vi "Oscilloscope.vi"() -> ()   [LabVIEW 2018]
doc: "This is a PC based 8-Channel Oscilloscope designed as a virtual instrument. The hardware interface is developed using Arduino Nano.\n\n\nDeveloped by:\nTanmay Vilas Samak\nChinmay Vilas Samak"
uses:
  <vilib>/MakerHub/LINX/Public/Peripherals/Analog/Analog Read 1 Chan.vi
  <vilib>/MakerHub/LINX/Public/Peripherals/Analog/Analog Read N Chans.vi
  <vilib>/MakerHub/LINX/Private/Local IO/LinxAnalogRead.vi
  <vilib>/MakerHub/LINX/Public/Utilities/Check Channel.vi
  <vilib>/MakerHub/LINX/Public/Utilities/Open Serial.vi
  <vilib>/MakerHub/LINX/Private/Utilties/Generate Error.vi
  <vilib>/MakerHub/LINX/LMH-LINX.lvlib
panel:
  out "CH8":bool
  out "CH7":bool
  out "CH6":bool
  out "CH5":bool
  out "CH4":bool
  out "CH3":bool
  out "CH2":bool
  out "CH1":bool
  in  "CH8":bool
  in  "CH7":bool
  in  "PAUSE":bool
  in  "Radio Buttons":T1(radio)
  in  "Save Image Button":bool
  in  "File Type":T1(radio)
  in  "Record & Stop Button":bool
  out "Record Time":dbl
  in  "Serial Port":refnum<visa-resource-name>="N/A"
  in  "POWER":bool
  in  "VOLTAGE DIVISION":i32(knob) scale=0.0..4.0
  in  "TIME DIVISION":i32(knob) scale=0.0..4.0
  in  "CH6":bool
  in  "CH5":bool
  in  "CH4":bool
  in  "CH3":bool
  in  "CH2":bool
  in  "CH1":bool
  out "Oscilloscope":T2(graph)
  # "OSCILLOSCOPE"
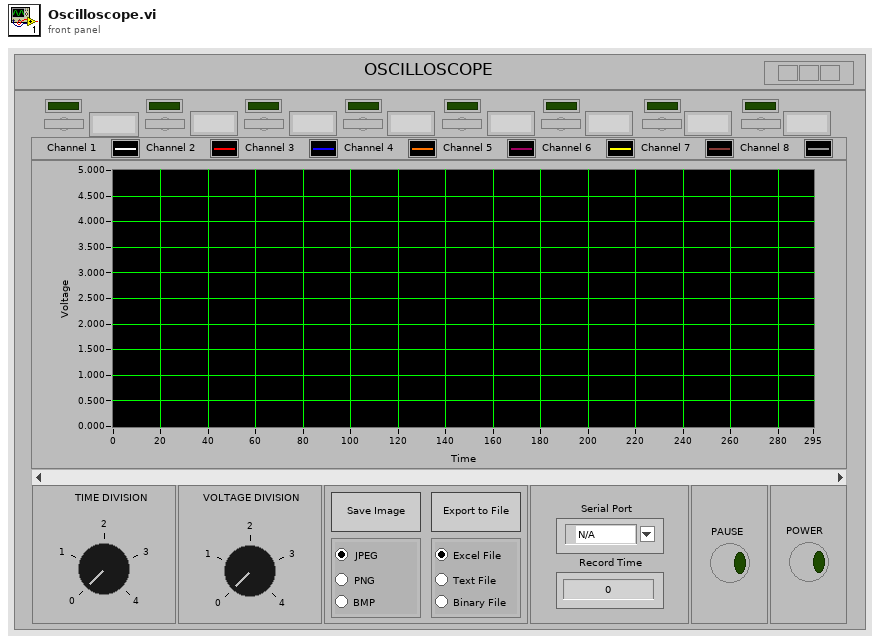
[diagram p1: front panel]
types:
  T1 = enum32{"Radio Selection 1", "Radio Selection 2", "Radio Selection 3"}
  T2 = cluster{"Voltage":dbl, "Voltage":dbl, "Voltage":dbl, "Voltage":dbl, "Voltage":dbl, "Voltage":dbl, "Voltage":dbl, "Voltage":dbl}
  T3 = cluster{"Voltage":dbl, "Voltage":dbl, "Voltage":dbl, "Voltage":dbl, "Voltage":dbl, "Voltage":dbl, "Voltage":dbl, "Voltage":dbl}[]
  T4 = enum8{"Enabled", "Disabled", "Disabled and Grayed Out"}
  T5 = typedef "LMH-LINX.lvlib/LINX Ref.ctl" = cluster{"IO":T6, "Interface":T7, "LINX Device Config":T8}
  T6 = typedef "LMH-LINX.lvlib/Platform.ctl" = enum16{"Remote", "Local"}
  T7 = typedef "LMH-LINX.lvlib/Interface.ctl" = enum16{"Serial", "TCP"}
  T8 = typedef "LMH-LINX.lvlib/Device.lvlib/LINX Device Config.ctl" = cluster{"Interface":T7, "COM Port":refnum<visa-resource-name>, "TCP Configuration":T9, "Device Family":u8, "Device ID":u8, "Device Name":string, "TCP Ref":refnum<k5>, "Channels":T10}
  T9 = typedef "LMH-LINX.lvlib/Device.lvlib/TCP Config.ctl" = cluster{"IP Address":string, "Port":u16}
  T10 = typedef "LMH-LINX.lvlib/Channels.ctl" = cluster{"DI":u8[], "DO":u8[], "AI":u8[], "AO":u8[], "PWM":u8[], "QE":u8[], "UART":u8[], "I2C 2":u8[], "SPI":u8[], "CAN":u8[], "Servo":u8[], "AI Ref (V)":dbl, "AI Resolution (Bits)":u8, "AO Ref (V)":dbl, "AO Resolution (Bits)":u8}
  T11 = typedef "imagedata.ctl" = cluster{"image type":i32, "image depth":i32, "image":u8[], "mask":u8[], "colors":u32[], "Rectangle":cluster{"left":i16, "top":i16, "right":i16, "bottom":i16}}
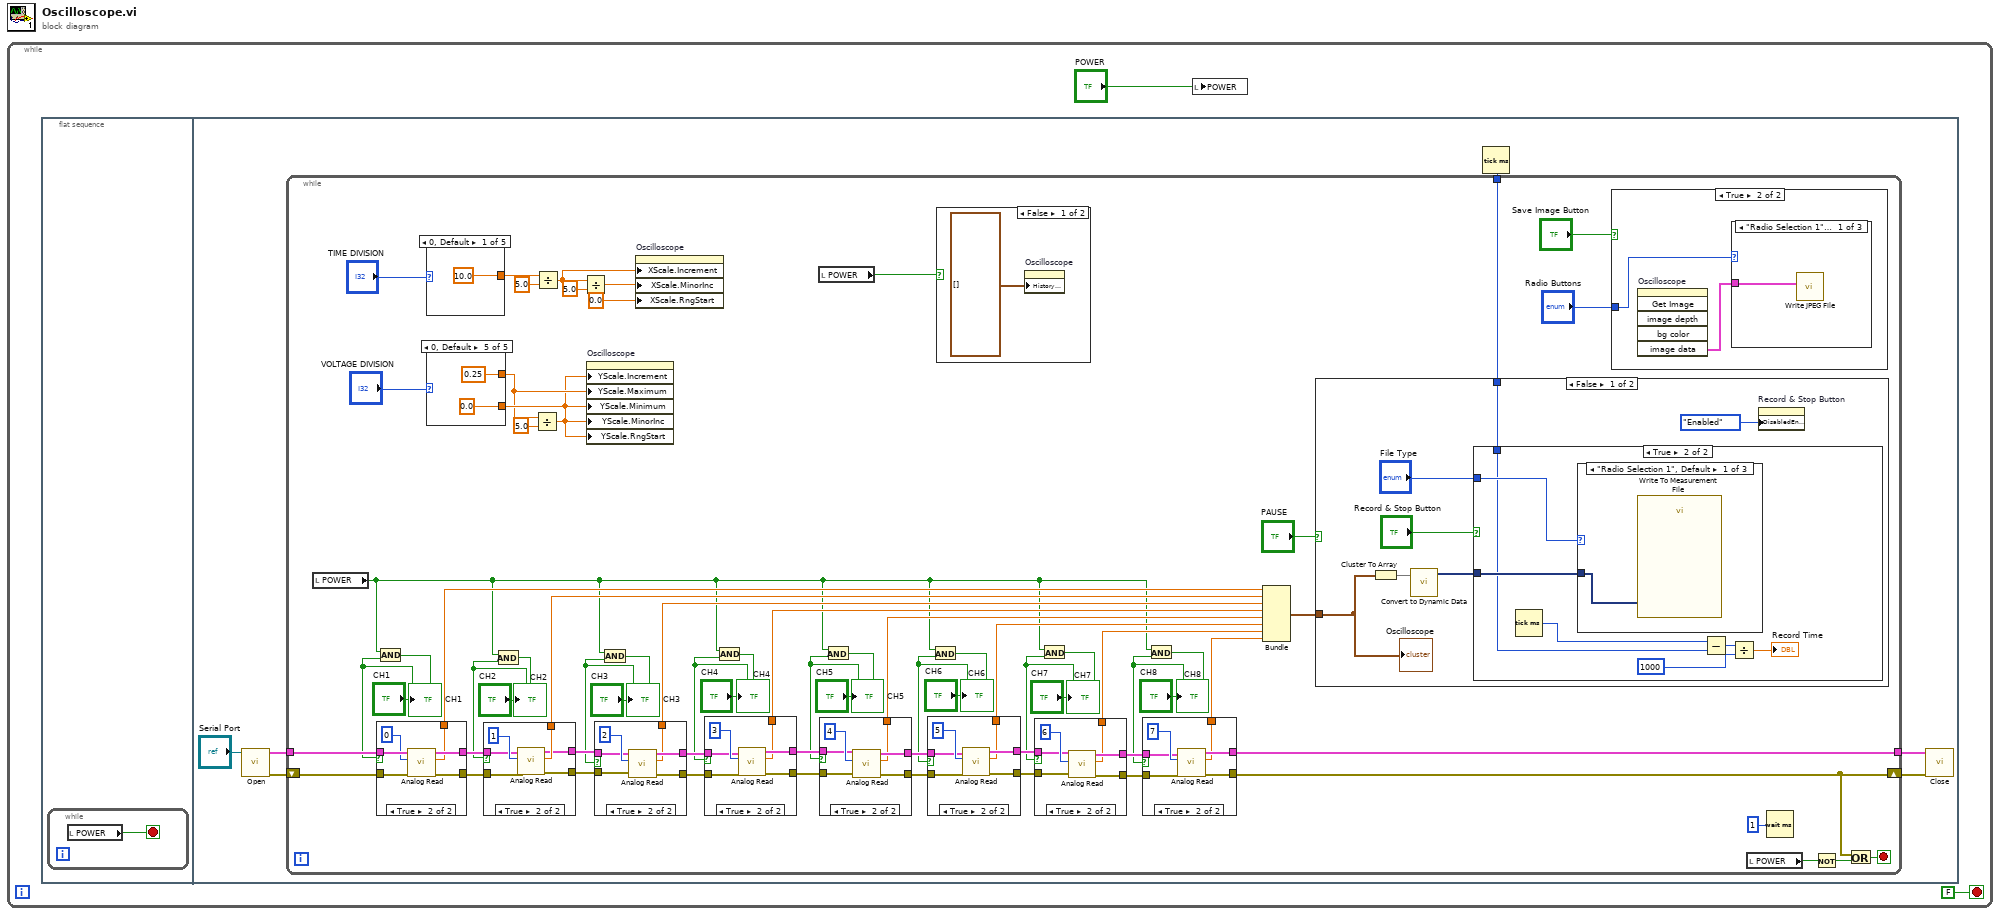
[diagram p0: block diagram]
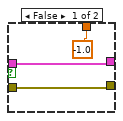
[diagram p3: hidden frame]
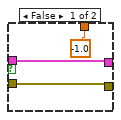
[diagram p4: hidden frame]
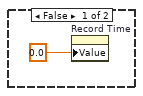
[diagram p5: hidden frame]
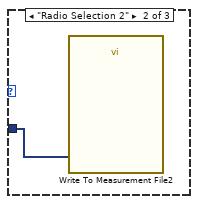
[diagram p6: hidden frame]
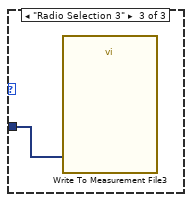
[diagram p7: hidden frame]
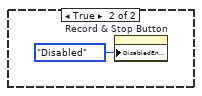
[diagram p8: hidden frame]
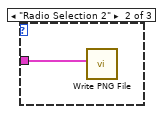
[diagram p10: hidden frame]
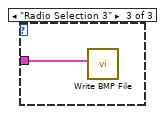
[diagram p11: hidden frame]
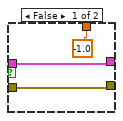
[diagram p12: hidden frame]
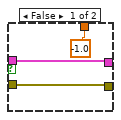
[diagram p13: hidden frame]
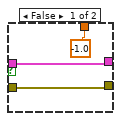
[diagram p14: hidden frame]
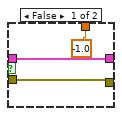
[diagram p15: hidden frame]
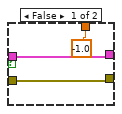
[diagram p16: hidden frame]
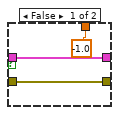
[diagram p17: hidden frame]
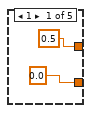
[diagram p18: hidden frame]
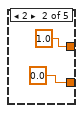
[diagram p19: hidden frame]
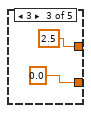
[diagram p20: hidden frame]
diagram:
  n1 = while {
    stop <- FALSE stop-if-true
    n2 = flat-sequence {
      frame #0 {
        n3 = while {
          stop <- w3 stop-if-true
          n4 = local read "POWER"() -> (w3:bool)
        }
      }
      frame #1 {
        n5 = call-poly <vilib>:"Open.vi"("Serial Port"="Serial Port") -> ("Error Out"=w7:errorcluster, "LINX Resource"=w6:T5)  [unwired: 8 in, 1 out]
        n6 = Tick Count (ms)() -> (millisecond timer value=w4:u32)
        n7 = while {
          shift-right: [w31] -> w9
          shift-left: w7 -> [w71]
          tunnel: w6 -> [w72]
          tunnel: [w32] -> w8
          tunnel: w4 -> [w38]
          stop <- w73 stop-if-true
          n8 = local read "POWER"() -> (w10:bool)
          n9 = case shown="True" "CH1" {
            tunnel: w72 -> [w165 w171]
            tunnel: w71 -> [w164 w170]
            tunnel: [w165 w168] -> w57
            tunnel: [w164 w167] -> w56
            tunnel: [-1.0 ("Voltage") w166] -> w55
            frame False {
            }
            frame True {
              n10 = call-poly <vilib>:"Analog Read.vi"("Error In"=w170, "Analog Channel"=u8 0 ("Channel 1 Pin"), "LINX Resource"=w171) -> ("Error Out"=w167:errorcluster, "Voltage"=w166:dbl, "LINX Resource"=w168:T5)  [unwired: 5 in, 1 out]
            }
          }
          n11 = And(x=w10, y="CH1") -> (x .and. y?=→"CH1":bool)
          n12 = case shown="0, Default" "TIME DIVISION" {
            tunnel: [10.0 20.0 50.0 100.0 200.0] -> w60
            frame 0, Default {
            }
            frame 1 {
            }
            frame 2 {
            }
            frame 3 {
            }
            frame 4 {
            }
          }
          n13 = case shown="0, Default" "VOLTAGE DIVISION" {
            tunnel: [0.5 1.0 2.5 5.0 0.25] -> w67
            tunnel: [0.0 0.0 0.0 0.0 0.0] -> w68
            frame 1 {
            }
            frame 2 {
            }
            frame 3 {
            }
            frame 4 {
            }
            frame 0, Default {
            }
          }
          n14 = case shown="True" "CH2" {
            tunnel: w57 -> [w155 w161]
            tunnel: w56 -> [w156 w160]
            tunnel: [-1.0 ("Voltage") w159] -> w54
            tunnel: [w156 w158] -> w51
            tunnel: [w155 w157] -> w42
            frame False {
            }
            frame True {
              n15 = call-poly <vilib>:"Analog Read.vi"("Error In"=w160, "Analog Channel"=u8 1 ("Channel 2 Pin"), "LINX Resource"=w161) -> ("Error Out"=w158:errorcluster, "Voltage"=w159:dbl, "LINX Resource"=w157:T5)  [unwired: 5 in, 1 out]
            }
          }
          n16 = And(x=w10, y="CH2") -> (x .and. y?=→"CH2":bool)
          n17 = Divide(x=w67, y=5.0) -> (x/y=w66:dbl)
          n18 = Divide(x=w60, y=5.0) -> (x/y=w62:dbl)
          n19 = Divide(x=w62, y=5.0) -> (x/y=w59:dbl)
          n20 = property on="Oscilloscope" class="WFChart (strict)"("YScale.Increment"=w66, "YScale.Maximum"=w67, "YScale.Minimum"=w68, "YScale.MinorInc"=w66, "YScale.RngStart"=w68) -> ()  [unwired: 2 in, 2 out]
          n21 = case shown="True" "CH3" {
            tunnel: [w147 w152] -> w53
            tunnel: [w146 w151] -> w52
            tunnel: w42 -> [w147 w150]
            tunnel: w51 -> [w146 w149]
            tunnel: [-1.0 ("Voltage") w148] -> w46
            frame False {
            }
            frame True {
              n22 = call-poly <vilib>:"Analog Read.vi"("Error In"=w149, "Analog Channel"=u8 2 ("Channel 3 Pin"), "LINX Resource"=w150) -> ("Error Out"=w151:errorcluster, "Voltage"=w148:dbl, "LINX Resource"=w152:T5)  [unwired: 5 in, 1 out]
            }
          }
          n23 = And(x=w10, y="CH3") -> (x .and. y?=→"CH3":bool)
          n24 = property on="Oscilloscope" class="WFChart (strict)"("XScale.Increment"=w62, "XScale.MinorInc"=w59, "XScale.RngStart"=0.0 ("X Scale.Range:Minimum")) -> ()  [unwired: 2 in, 2 out]
          n25 = case shown="True" "CH4" {
            tunnel: w53 -> [w138 w143]
            tunnel: w52 -> [w137 w142]
            tunnel: [w138 w141] -> w48
            tunnel: [w137 w140] -> w47
            tunnel: [-1.0 ("Voltage") w139] -> w45
            frame False {
            }
            frame True {
              n26 = call-poly <vilib>:"Analog Read.vi"("Error In"=w142, "Analog Channel"=u8 3 ("Channel 4 Pin"), "LINX Resource"=w143) -> ("Error Out"=w140:errorcluster, "Voltage"=w139:dbl, "LINX Resource"=w141:T5)  [unwired: 5 in, 1 out]
            }
          }
          n27 = And(x=w10, y="CH4") -> (x .and. y?=→"CH4":bool)
          n28 = local read "POWER"() -> (w25:bool)
          n29 = case shown="True" "CH5" {
            tunnel: [w129 w134] -> w50
            tunnel: [w128 w133] -> w49
            tunnel: w48 -> [w129 w132]
            tunnel: w47 -> [w128 w131]
            tunnel: [-1.0 ("Voltage") w130] -> w44
            frame False {
            }
            frame True {
              n30 = call-poly <vilib>:"Analog Read.vi"("Error In"=w131, "Analog Channel"=u8 4 ("Channel 5 Pin"), "LINX Resource"=w132) -> ("Error Out"=w133:errorcluster, "Voltage"=w130:dbl, "LINX Resource"=w134:T5)  [unwired: 5 in, 1 out]
            }
          }
          n31 = And(x=w10, y="CH5") -> (x .and. y?=→"CH5":bool)
          n32 = case shown="True" "CH6" {
            tunnel: w50 -> [w120 w125]
            tunnel: w49 -> [w119 w124]
            tunnel: [w120 w123] -> w34
            tunnel: [w119 w122] -> w33
            tunnel: [-1.0 ("Voltage") w121] -> w43
            frame False {
            }
            frame True {
              n33 = call-poly <vilib>:"Analog Read.vi"("Error In"=w124, "Analog Channel"=u8 5 ("Channel 6 Pin"), "LINX Resource"=w125) -> ("Error Out"=w122:errorcluster, "Voltage"=w121:dbl, "LINX Resource"=w123:T5)  [unwired: 5 in, 1 out]
            }
          }
          n34 = And(x=w10, y="CH6") -> (x .and. y?=→"CH6":bool)
          n35 = case shown="False" w25 {
            frame False {
              n36 = property on="Oscilloscope" class="WFChart (strict)"("History Data"=T3 []) -> ()  [unwired: 2 in, 2 out]
            }
            frame True {
            }
          }
          n37 = case shown="True" "CH7" {
            tunnel: [w87 w92] -> w36
            tunnel: [w86 w91] -> w35
            tunnel: w34 -> [w87 w90]
            tunnel: w33 -> [w86 w89]
            tunnel: [-1.0 ("Voltage") w88] -> w30
            frame False {
            }
            frame True {
              n38 = call-poly <vilib>:"Analog Read.vi"("Error In"=w89, "Analog Channel"=u8 6 ("Channel 5 Pin"), "LINX Resource"=w90) -> ("Error Out"=w91:errorcluster, "Voltage"=w88:dbl, "LINX Resource"=w92:T5)  [unwired: 5 in, 1 out]
            }
          }
          n39 = And(x=w10, y="CH7") -> (x .and. y?=→"CH7":bool)
          n40 = case shown="True" "CH8" {
            tunnel: w36 -> [w78 w83]
            tunnel: w35 -> [w77 w82]
            tunnel: [w78 w81] -> w32
            tunnel: [w77 w80] -> w31
            tunnel: [-1.0 ("Voltage") w79] -> w29
            frame False {
            }
            frame True {
              n41 = call-poly <vilib>:"Analog Read.vi"("Error In"=w82, "Analog Channel"=u8 7 ("Channel 6 Pin"), "LINX Resource"=w83) -> ("Error Out"=w80:errorcluster, "Voltage"=w79:dbl, "LINX Resource"=w81:T5)  [unwired: 5 in, 1 out]
            }
          }
          n42 = And(x=w10, y="CH8") -> (x .and. y?=→"CH8":bool)
          n43 = Bundle("Voltage"=w55, "Voltage"=w54, "Voltage"=w46, "Voltage"=w45, "Voltage"=w44, "Voltage"=w43, "Voltage"=w30, "Voltage"=w29) -> (w41:T2)  [unwired: 1 in]
          n44 = case shown="False" "PAUSE" {
            tunnel: w41 -> [w95 _]
            tunnel: w38 -> [w96 _]
            frame False {
              n45 = Cluster To Array(cluster=w95) -> (array=w97:dbl[])
              n46 = call "Convert to Dynamic Data"("Array"=w97) -> ("Dynamic Data Type"=w100:dynamicdata)  [unwired: 3 in]
              n47 = case shown="True" "Record & Stop Button" {
                tunnel: w100 -> [_ w108]
                tunnel: w96 -> [_ w102]
                tunnel: "File Type" -> [_ w104]
                frame False {
                  n48 = property on="Record Time" class="DigNum (strict)"("Value"=0.0 ("Recorded time")) -> ()  [unwired: 2 in, 2 out]
                }
                frame True {
                  n49 = Tick Count (ms)() -> (millisecond timer value=w103:u32)
                  n50 = case shown="\"Radio Selection 1\", Default" w104 {
                    tunnel: w108 -> [w109 w110 w111]
                    frame "Radio Selection 1", Default {
                      n51 = call "Write To Measurement File"("Signals"=w109) -> ()  [unwired: 16 in, 3 out]
                    }
                    frame "Radio Selection 2" {
                      n52 = call "Write To Measurement File2"("Signals"=w110) -> ()  [unwired: 16 in, 3 out]
                    }
                    frame "Radio Selection 3" {
                      n53 = call "Write To Measurement File3"("Signals"=w111) -> ()  [unwired: 16 in, 3 out]
                    }
                  }
                  n54 = Subtract(x=w103, y=w102) -> (x-y=w107:u32)
                  n55 = Divide(x=w107, y=u32 1000) -> (x/y=→"Record Time":dbl)
                }
              }
              n56 = property on="Record & Stop Button" class="Bool (strict)"("DisabledEnum"=T4."Enabled" ("Disabled")) -> ()  [unwired: 2 in, 2 out]
              "Oscilloscope" <- w95
            }
            frame True {
              n57 = property on="Record & Stop Button" class="Bool (strict)"("DisabledEnum"=T4."Disabled" ("Disabled")) -> ()  [unwired: 2 in, 2 out]
            }
          }
          n58 = case shown="True" "Save Image Button" {
            tunnel: "Radio Buttons" -> [_ w113]
            frame False {
            }
            frame True {
              n59 = invoke on="Oscilloscope" class="WFChart (strict)" method="Get Image"() -> ("image data"=w114:T11)  [unwired: 6 in, 5 out]
              n60 = case shown="\"Radio Selection 1\", Default" w113 {
                tunnel: w114 -> [w115 w116 w117]
                frame "Radio Selection 1", Default {
                  n61 = call <vilib>:"Write JPEG File.vi"("image data"=w115) -> ()  [unwired: 9 in, 2 out]
                }
                frame "Radio Selection 2" {
                  n62 = call <vilib>:"Write PNG File.vi"("image data"=w116) -> ()  [unwired: 9 in, 2 out]
                }
                frame "Radio Selection 3" {
                  n63 = call <vilib>:"Write BMP File.vi"("image data"=w117) -> ()  [unwired: 9 in, 2 out]
                }
              }
            }
          }
          n64 = local read "POWER"() -> (w28:bool)
          n65 = Wait (ms)(milliseconds to wait=u32 1) -> ()  [unwired: 1 out]
          n66 = Not(x=w28) -> (.not. x?=w58:bool)
          n67 = Or(x=w31, y=w58) -> (x .or. y?=w73:bool)
        }
        n68 = call <vilib>:"Close.vi"("Error In"=w9, "LINX Resource"=w8) -> ()  [unwired: 9 in, 1 out]
      }
    }
    n69 = local write "POWER"("POWER") -> ()
  }
